vi "GET_COUNTER.vi"(3 "reset":bool, 4 "Option Edge":dbl=1.0, 5 "error in (no error)":errorcluster, 6 "VISA resource name":refnum<visa-resource-name>) -> (0 "count":u8, 1 "error out":errorcluster, 2 "VISA resource Salida":refnum<visa-resource-name>)   [LabVIEW 2011]
panel:
  out "unsigned byte array":u8[](array[numeric])
  out "Read get_Counter command":u8[](array[numeric])
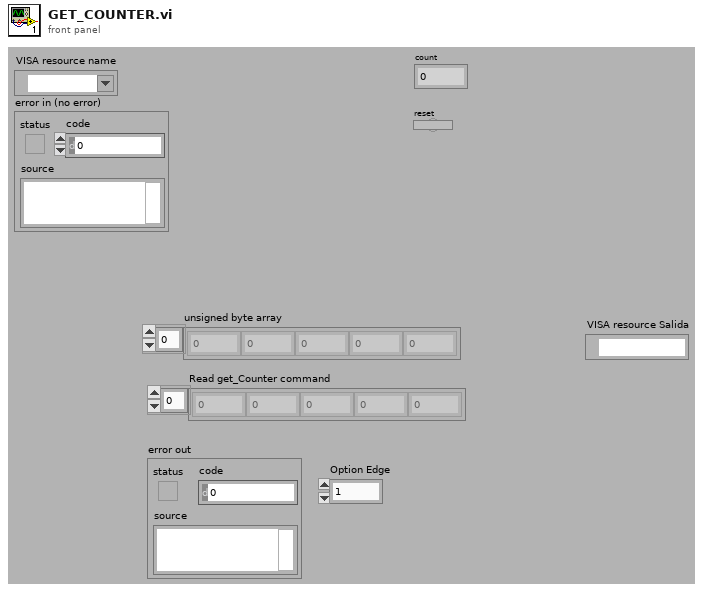
[diagram p1: front panel]
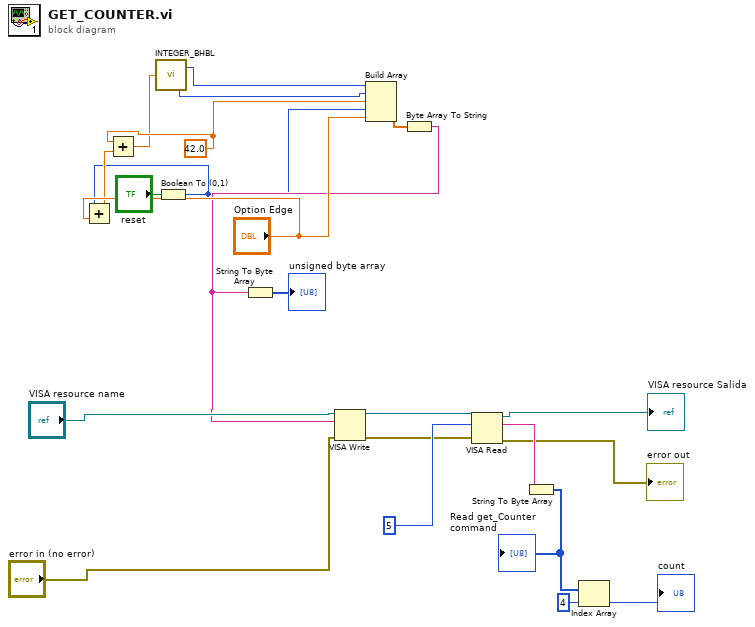
[diagram p0: block diagram]
diagram:
  w10 = 42.0 ("element")
  n1 = Boolean To (0,1)(Boolean="reset") -> (0, 1=w1:i16)
  n2 = Add(x=w1, y="Option Edge") -> (x+y=w11:dbl)
  n3 = Add(x=w10, y=w11) -> (x+y=w9:dbl)
  n4 = call "INTEGER_BHBL.vi"("int16"=w9) -> ("Lvalue"=w7:u8, "HValue"=w8:u8)
  n5 = Build Array(w8, w7, w10, w1, "Option Edge") -> (w16:dbl[])
  n6 = Byte Array To String(unsigned byte array=w16) -> (string=w6:string)
  n7 = String To Byte Array(string=w6) -> (unsigned byte array=→"unsigned byte array":u8[])
  n8 = VISA Write(VISA resource name="VISA resource name", write buffer=w6, error in (no error)="error in (no error)") -> (VISA resource name out=w17:refnum<visa-resource-name>, error out=w19:errorcluster)  [unwired: 1 out]
  n9 = VISA Read(VISA resource name=w17, byte count=u32 5, error in (no error)=w19) -> (VISA resource name out=→"VISA resource Salida":refnum<visa-resource-name>, read buffer=w21:string, error out=→"error out":errorcluster)  [unwired: 1 out]
  n10 = String To Byte Array(string=w21) -> (unsigned byte array=w4:u8[])
  "Read get_Counter command" <- w4
  n11 = Index Array(array=w4, index=4) -> (element=→"count":u8)
